vi "DataFinder Property Node.vi"   [LabVIEW 2020]
doc: "Provides properties that you use to configure the DataFinder."
uses:
  <resource>/objmgr/DataFinder.rc
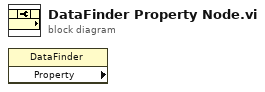
[diagram p0: block diagram]
diagram:
  n1 = property class="DataFinder" props=[]() -> ()  [unwired: 2 in, 3 out]
